vi "select gating.vi"() -> ()   [LabVIEW 2016]
doc: "Takes the pixie 4 values and creates a 2d spectrum based on the gate ROI and the desired spectrum"
uses:
  pixie2d/controls/energy 2d selection.ctl
  pixie2d/sub vi/chopper.ctl
  <vilib>/Utility/miscctls.llb/LVPointDoubleTypeDef.ctl
  controls/read write shift control.ctl
  <vilib>/DAQmx/write.llb/DAQmx Write (Digital Wfm 1Chan NSamp).vi
  <vilib>/Waveform/DWDTOps.llb/DWDT Uncompress Digital.vi
  <vilib>/DAQmx/miscellaneous.llb/DAQmx Fill In Error Info.vi
  <vilib>/Waveform/DWDTOps.llb/DWDT Boolean Array to Digital.vi
  <vilib>/DAQmx/configure/timing.llb/DAQmx Timing (Burst Import Clock).vi
  <vilib>/Waveform/DWDTOps.llb/DWDT Append Digital Samples.vi
  <resource>/objmgr/daqmx.rc
  <vilib>/Analysis/NI_AALPro.lvlib
panel:
  out "Chopper gain error":errorcluster
  in  "Tab Control":T1(tab)
  in  "stop":bool
  in  "set gate":bool
  in  "reset spectrum":bool
  in  "which spectrum":string(combo)="full spectrum pulser"
  in  "gate change":bool
  out "2d display":u64[][](graph) caption="full spectrum"
  in  "save image":bool
  out "2d gate active?":bool
  out "X Peak":i32
  out "Y peak":i32
  in  "na/V":dbl=1000.0
  in  "Energy 2d gate":T2="1 vs 2"
  in  "channel":string(combo)="Channel 1"
  out "MCA Histograms":u32[][](graph)
  in  "gain":i32=10 min=1 max=100 step=1
  in  "beam chopper":T3
  out "data":string
  out "task done?":bool
  out "location":dbl
  out "peak":dbl
  out "fwhm":i32
  in  "Module number":u16
  in  "reset count rate (cps)":i32=500000
  out "Loop iterations":i32
  out "std percent":dbl format="%0.2f"
  in  "chopper gain":i32(slide)=50 scale=0.0..20.0
  out "digital data out 3":digitaldata
  out "digital data out 2":digitaldata
  out "output waveform 3":digitalwaveform(waveform)={"t0"=timestamp(0 s since 1904-01-01), "dt"=1.0, "Y"={"transitions"=[], "data"=[]}}
  out "output waveform 2":digitalwaveform(waveform)={"t0"=timestamp(0 s since 1904-01-01), "dt"=1.0, "Y"={"transitions"=[], "data"=[]}}
  out "20UA_Chop_Tune.hws":digitalwaveform(waveform)={"t0"=timestamp(0 s since 1904-01-01), "dt"=1e-06, "Y"={"transitions"=[], "data"=array100000x16[1600000 elements]}}
  out "MCA Histogram cursor error":errorcluster
  out "Chopper error":errorcluster
  out "Tune Stable to Detector Error":errorcluster
  out "Chopper Pulse Creation error":errorcluster
  out "Chopped Current SV error":errorcluster
  out "DAQmx task end error 2":errorcluster
  out "DAQmx task end error 1":errorcluster
  out "Stop/Chopper Variant conversion":errorcluster
  out "Tune Stable DAQmx write error":errorcluster
  in  "chopper factor":u32(knob)=5 scale=0.0..10.0
  # "Directions\n1) select which spectrum \n     and 2d gate you want\n     to  view\n\n2)  When the ROI is located\n      double click on\n      chart to start\n      drawing gate\n\n3)   When gate is drawn,\n      double click the mouse to \n      stop the gate from being\n      drawn.  press gate \n       change and set gate will\n      appear\n\n4)   press set gate, and\n      gate will be generated\n\n5)  Once the gate is drawn,\n      make sure it covers the \n      region that you want\n      defined\n\n6)  To view gate, right click\n      on graph and select view\n     gates."
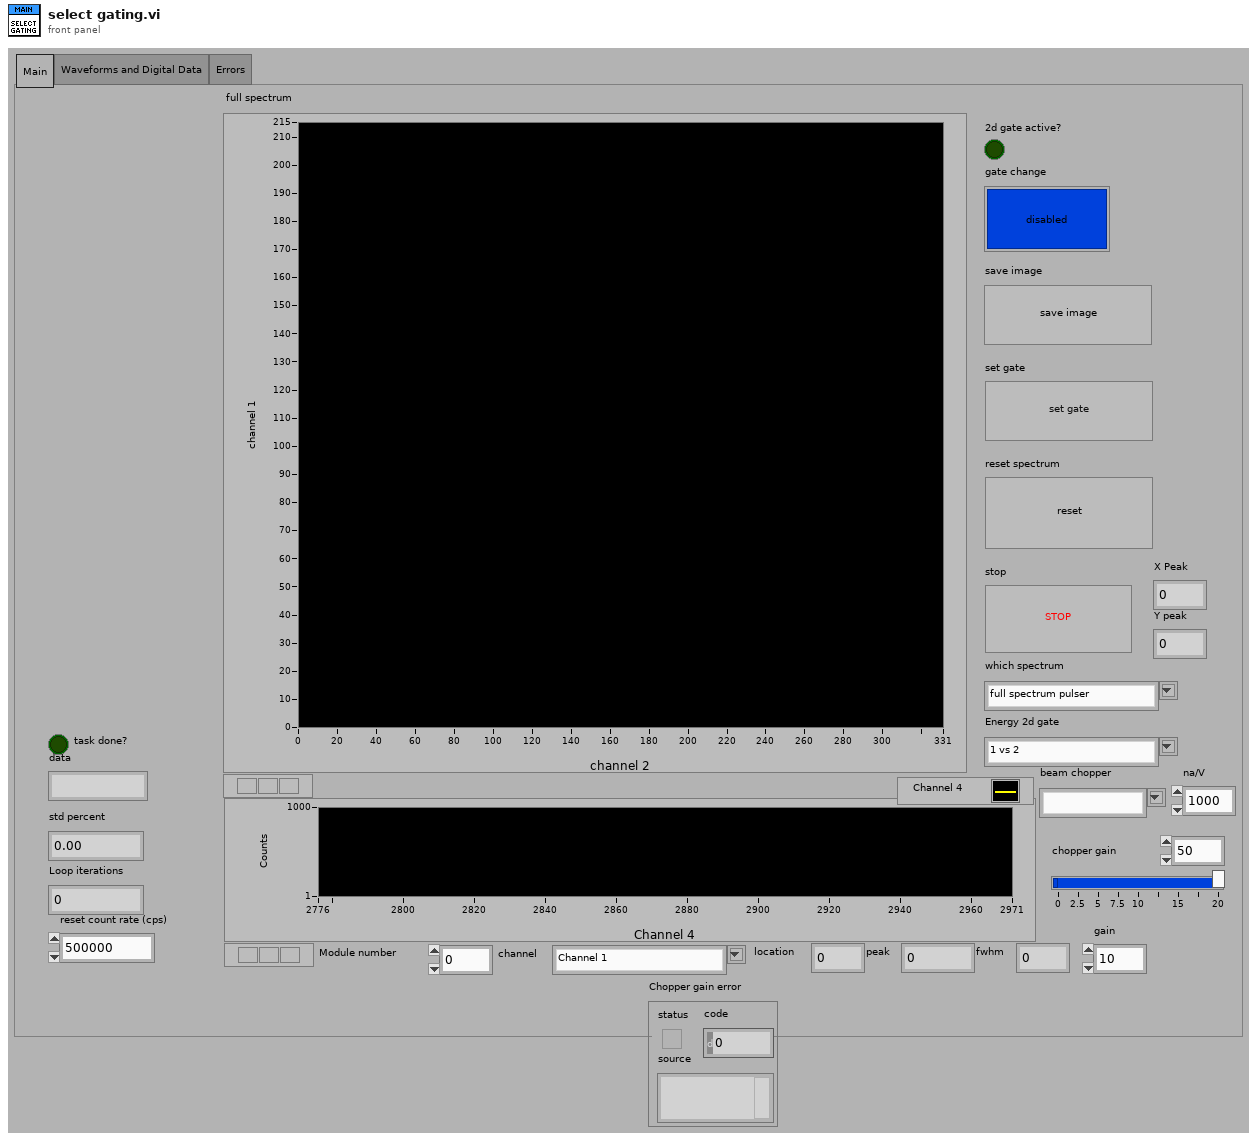
[diagram p1: front panel]
types:
  T1 = enum32{"Main", "Waveforms and Digital Data", "Errors"}
  T2 = typedef "energy 2d selection.ctl" = string
  T3 = typedef "chopper.ctl" = string
  T4 = typedef "LVPointDoubleTypeDef.ctl" = cluster{"X":dbl, "Y":dbl}
  T5 = typedef "read write shift control.ctl" = string
  T6 = typedef "LVPoint32TypeDef.ctl" = cluster{"Horizontal":i32, "Vertical":i32}
  T7 = typedef "imagedata.ctl" = cluster{"image type":i32, "image depth":i32, "image":u8[], "mask":u8[], "colors":u32[], "Rectangle":cluster{"left":i16, "top":i16, "right":i16, "bottom":i16}}
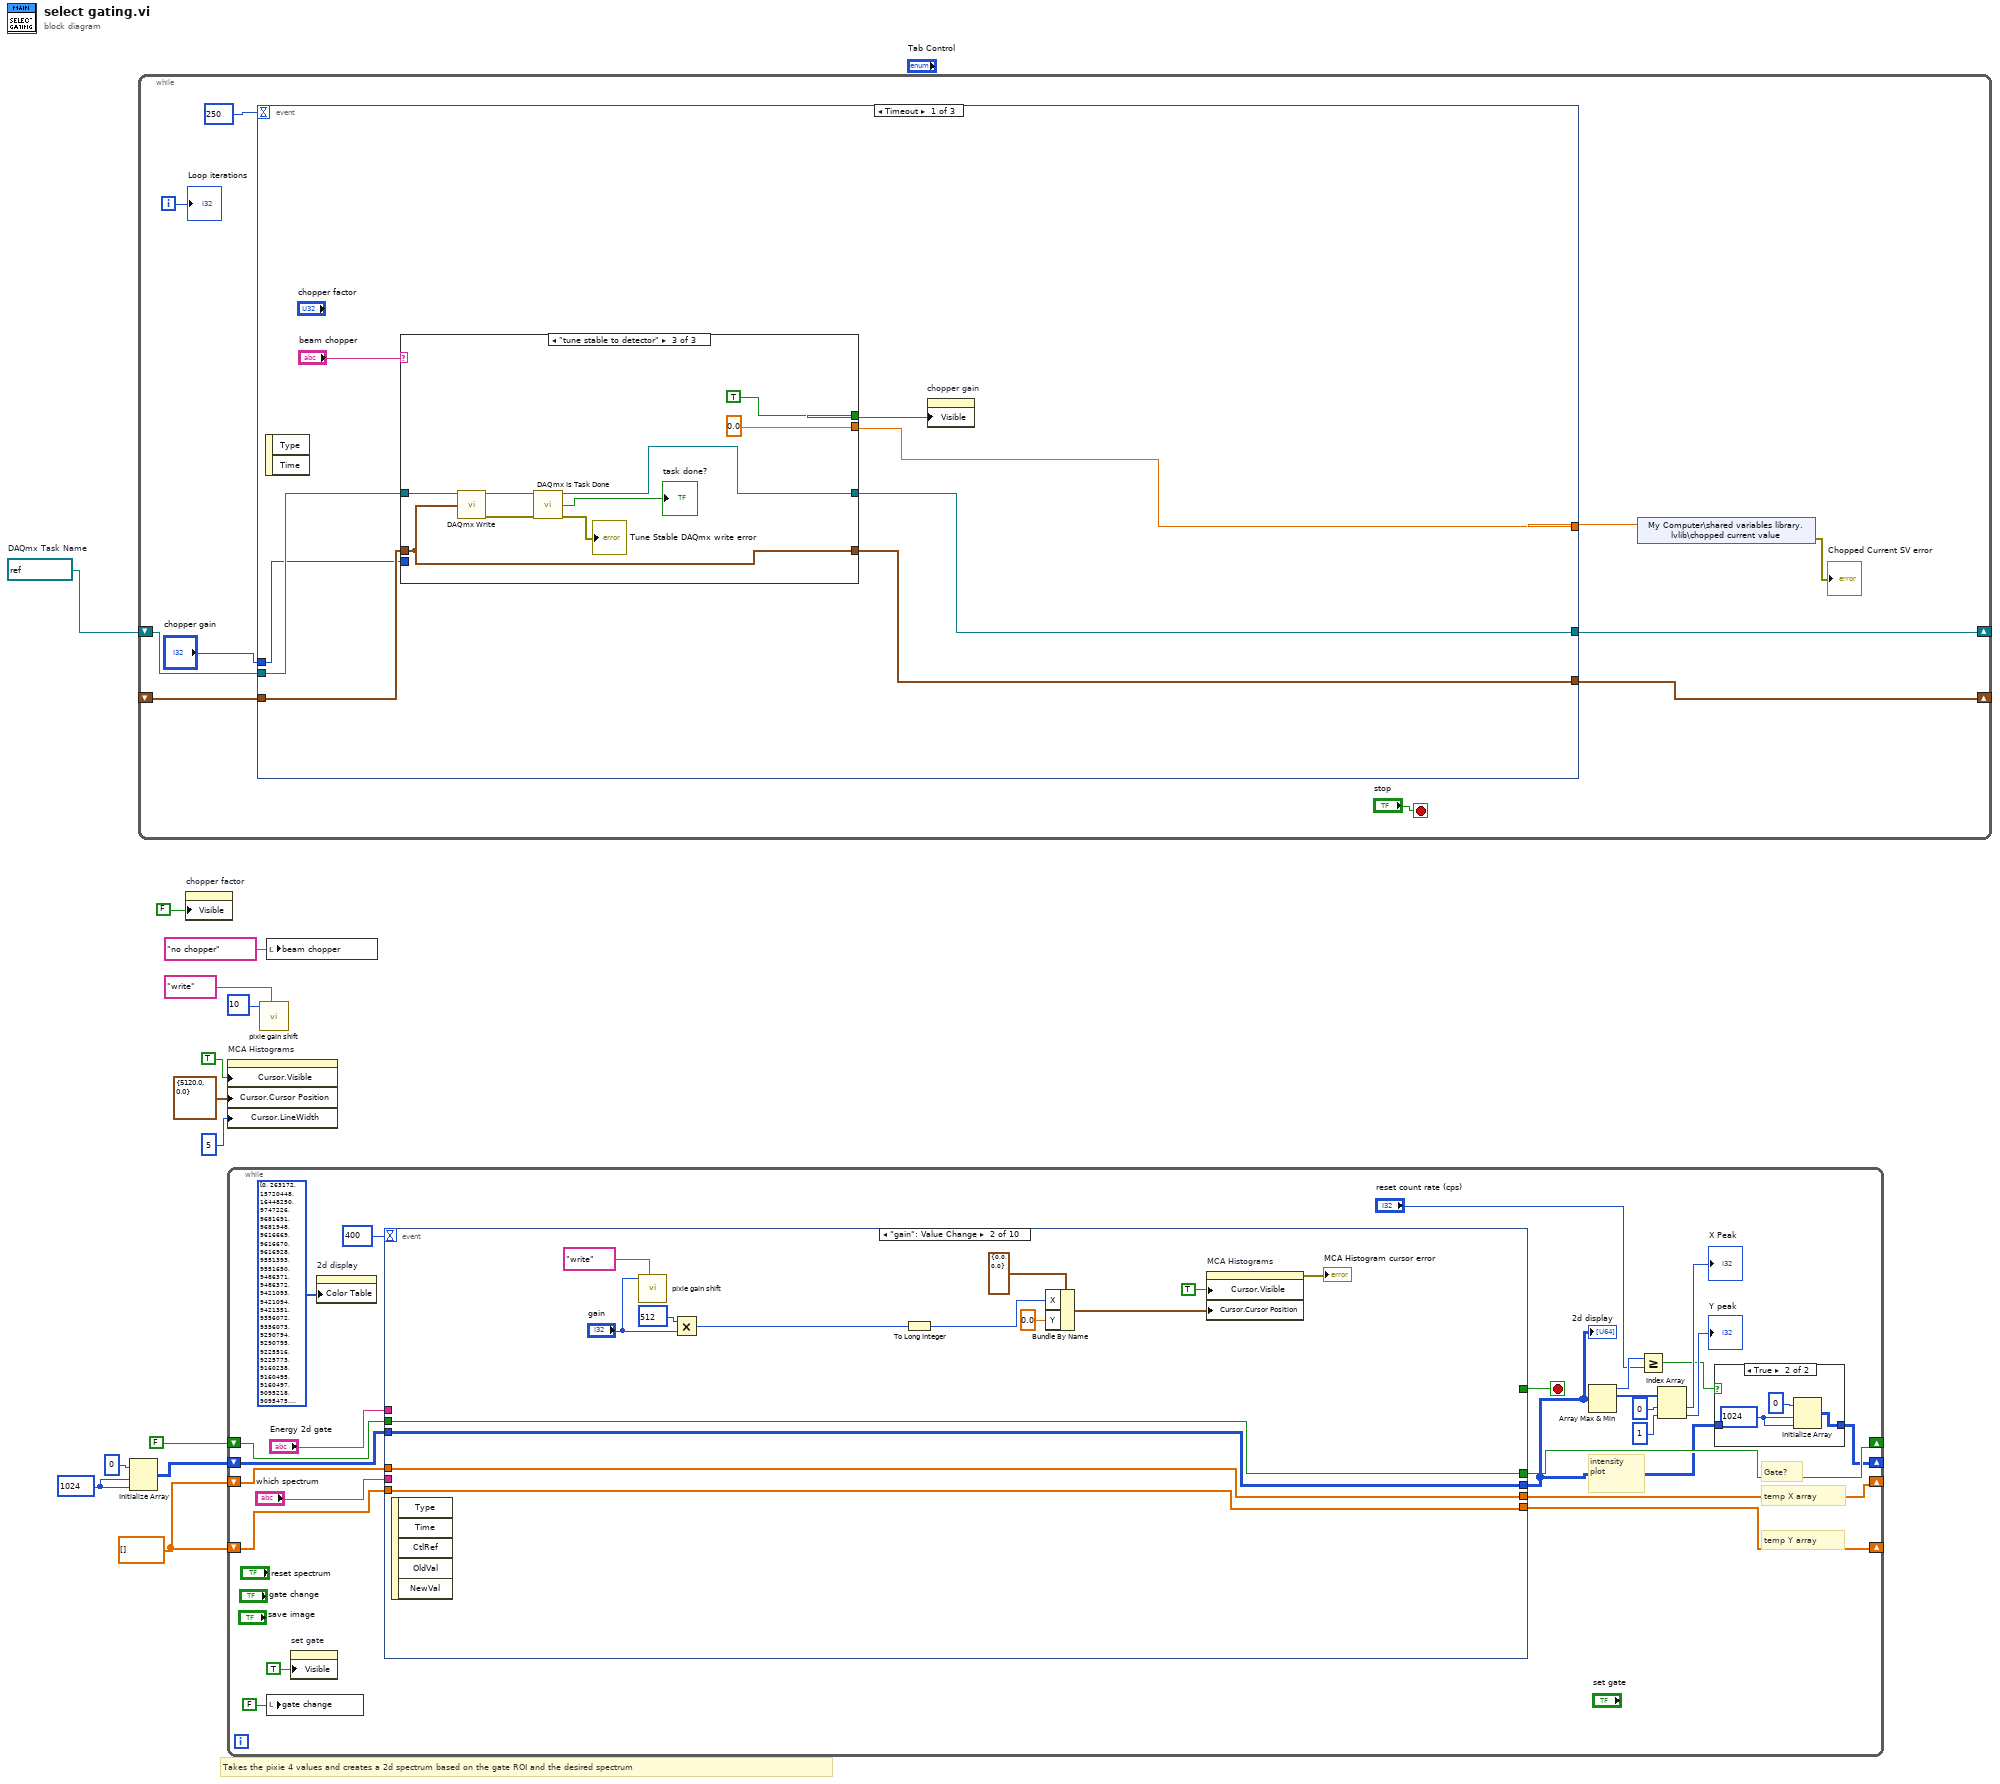
[diagram p0: block diagram]
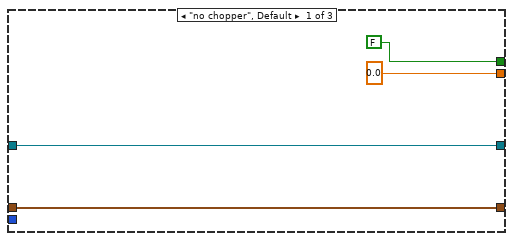
[diagram p2: hidden frame]
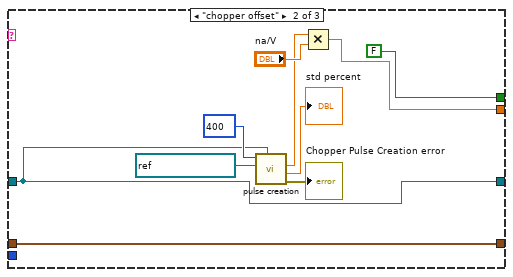
[diagram p3: hidden frame]
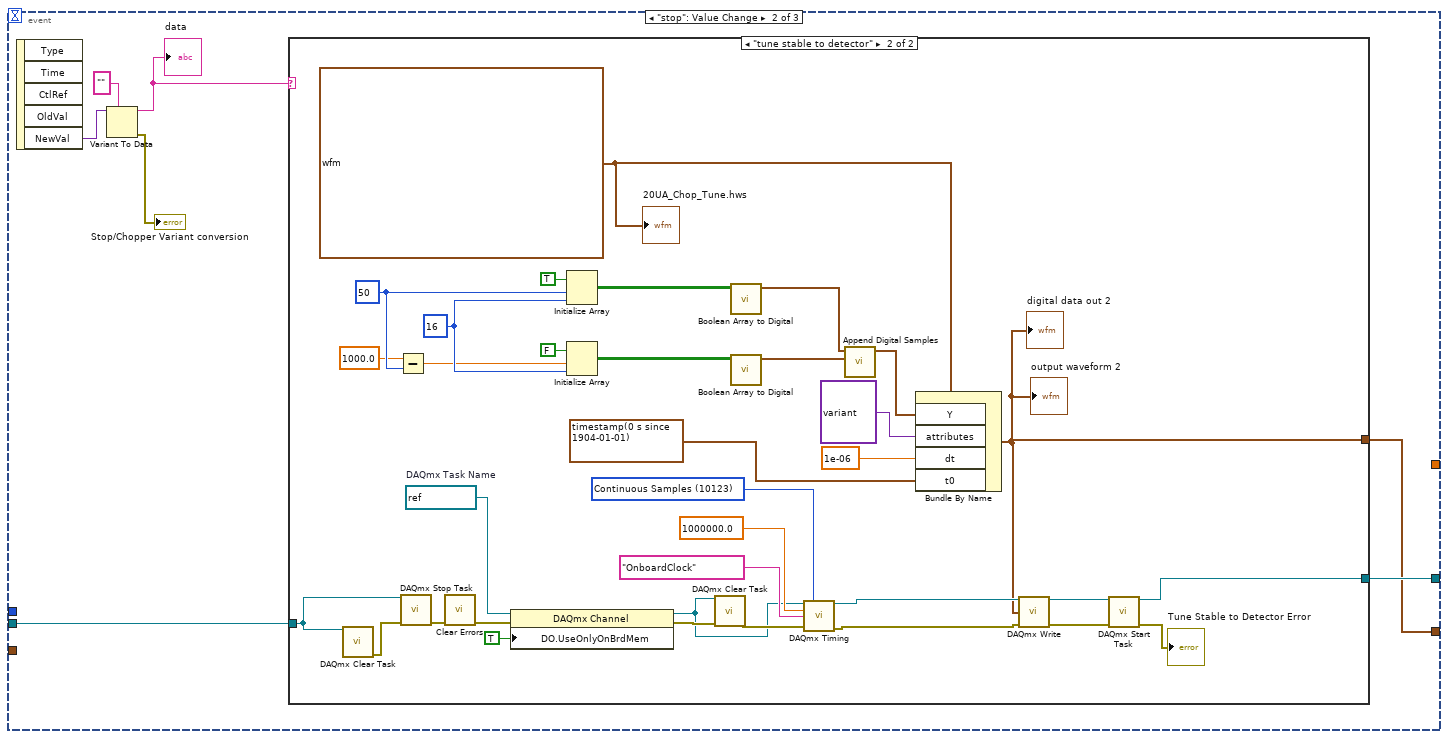
[diagram p4: hidden frame]
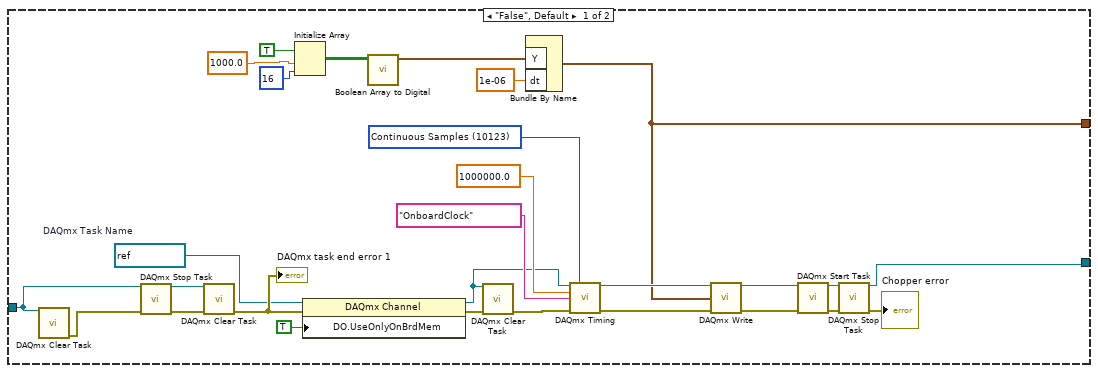
[diagram p5: hidden frame]
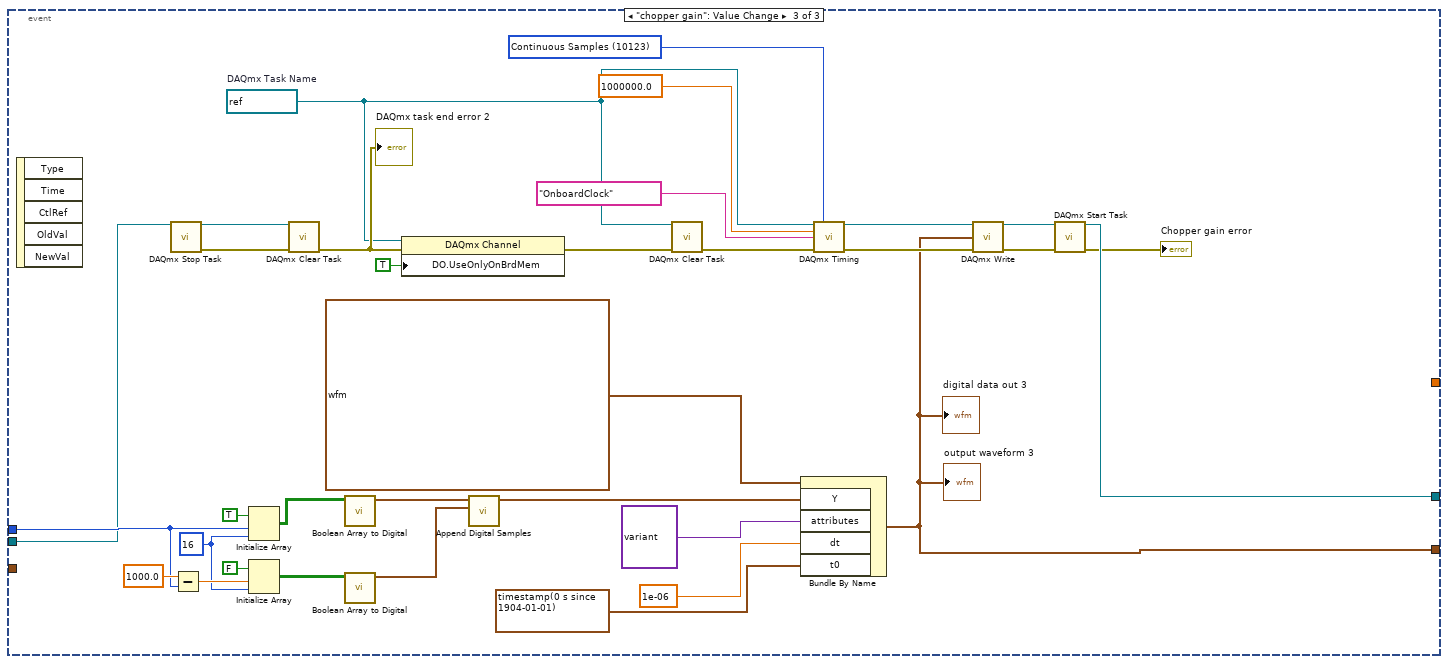
[diagram p6: hidden frame]
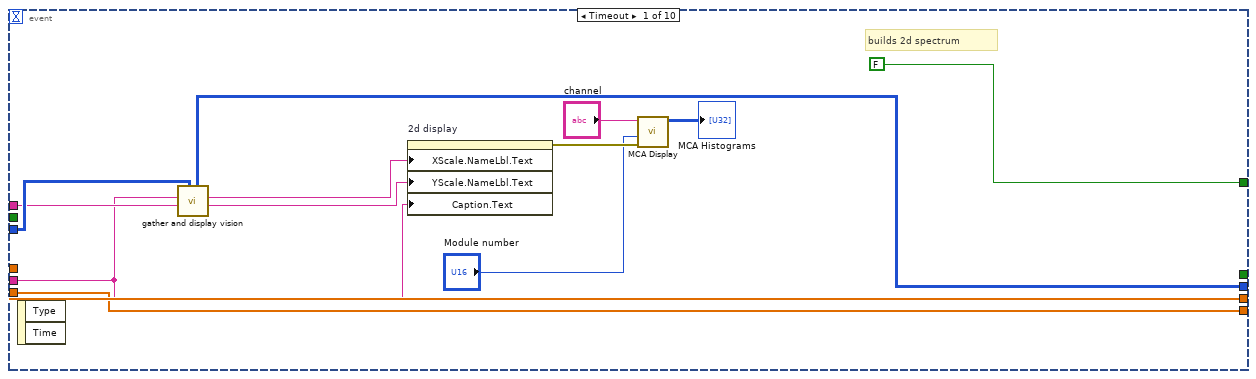
[diagram p8: hidden frame]
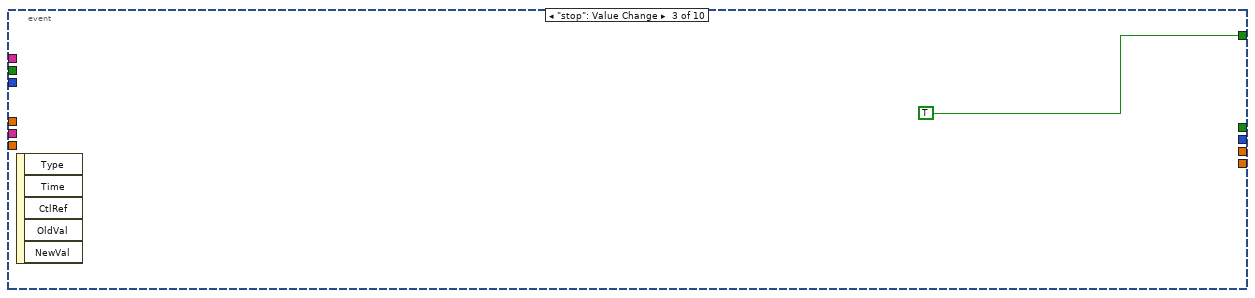
[diagram p9: hidden frame]
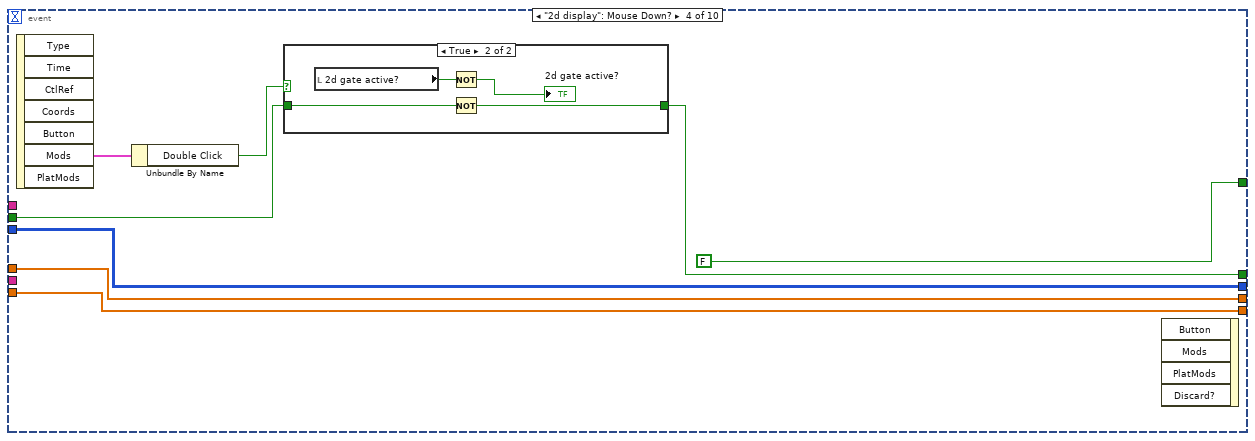
[diagram p10: hidden frame]
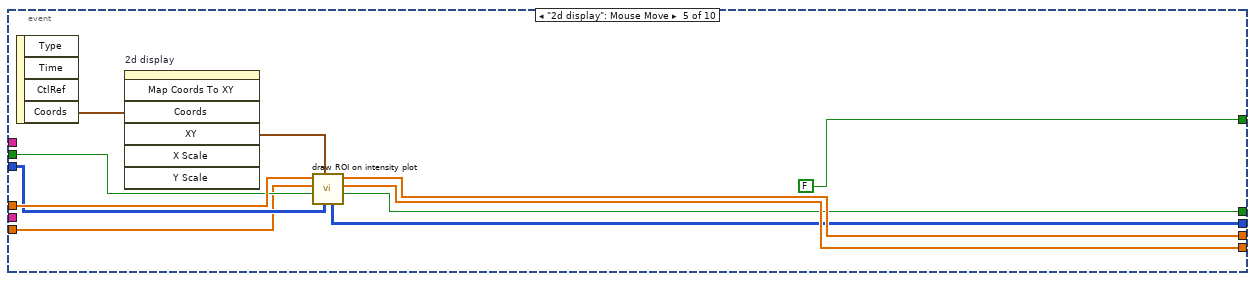
[diagram p12: hidden frame]
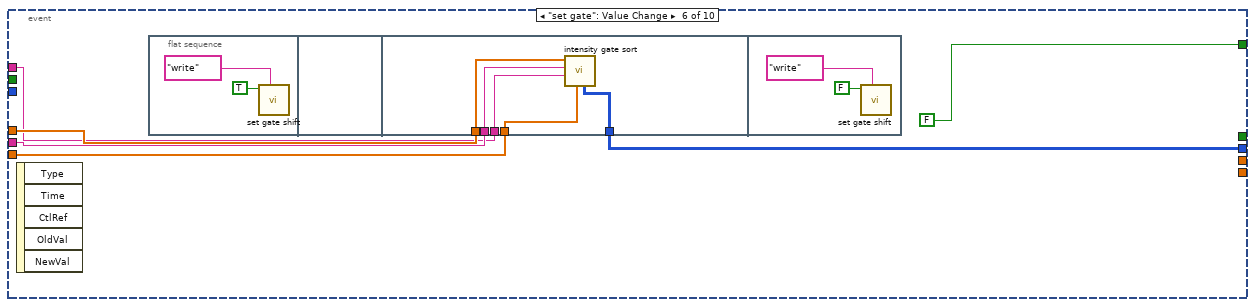
[diagram p13: hidden frame]
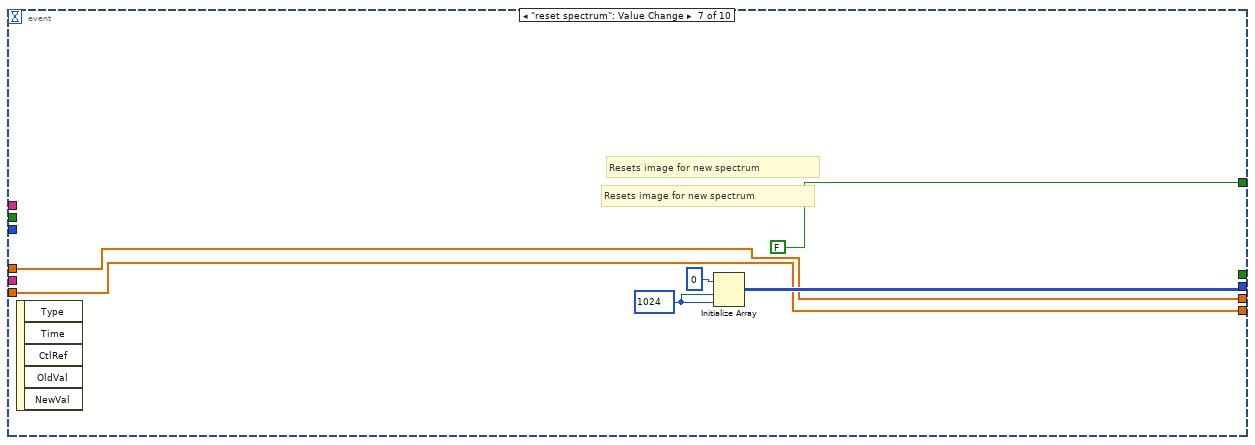
[diagram p14: hidden frame]
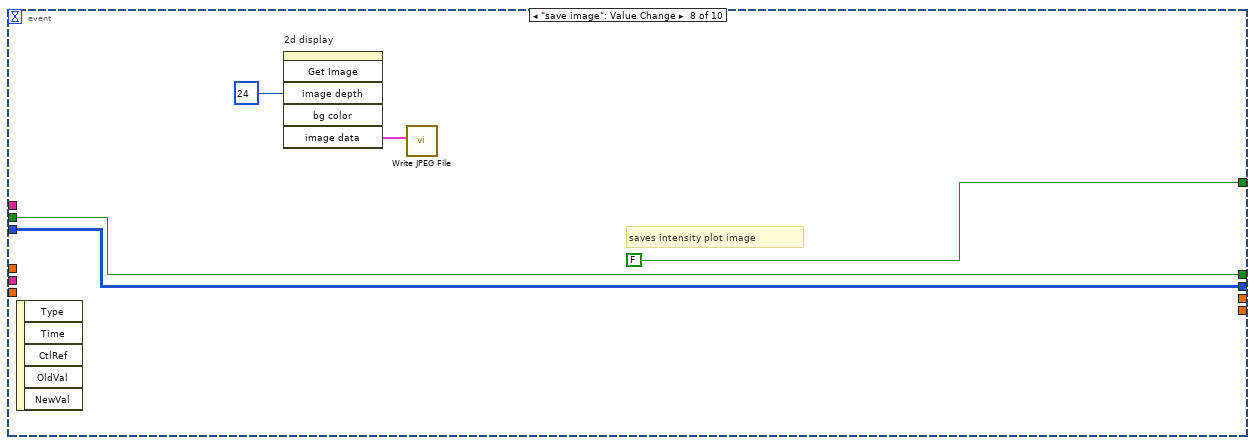
[diagram p15: hidden frame]
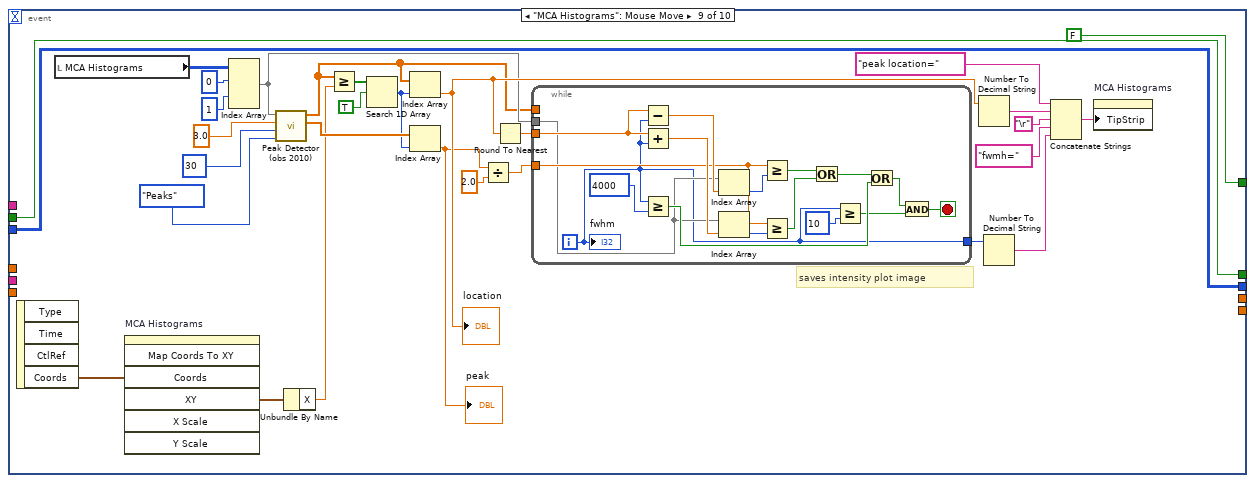
[diagram p16: hidden frame]
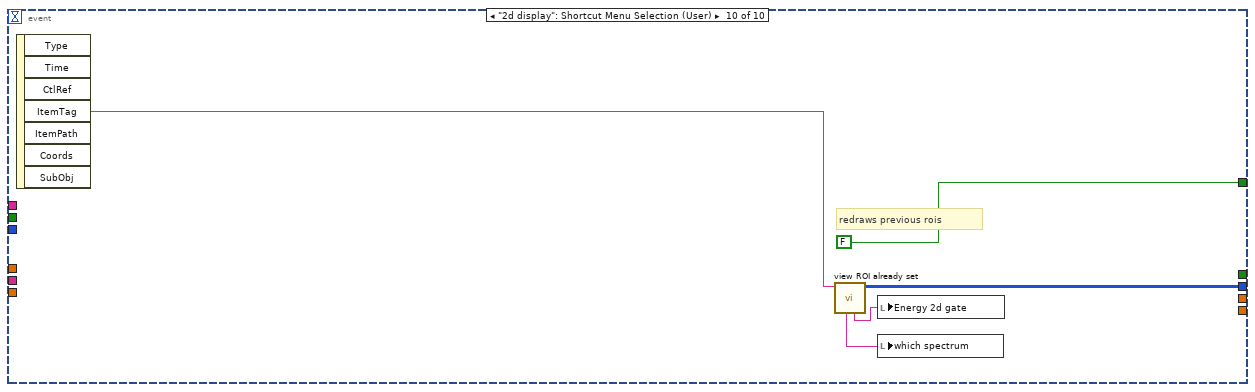
[diagram p17: hidden frame]
diagram:
  w1 = refnum<k21> "chop2"  # DAQmx Task Name
  w9 = dbl[] []
  w13 = u64 1024
  # "Takes the pixie 4 values and creates a 2d spectrum based on the gate ROI and the desired spectrum"
  n1 = Initialize Array(u64 0 ("X Resolution"), w13, w13) -> (w11:u64[][])
  n2 = while {
    shift-right: [w19] -> _
    shift-left: _ -> [w18]
    shift-right: [w16] -> _
    shift-left: w1 -> [w22]
    i -> [w15]
    stop <- "stop" stop-if-true
    n3 = event shown="[0] Timeout" {
      selector: _ -> [_ _ _]
      dyn-events: _ -> [_ _ _]
      timeout: 250 -> [_ _ _]
      tunnel: [w24 _ _] -> w23
      tunnel: w22 -> [w31 w58 w125]
      tunnel: [w29 w55 w128] -> w19
      tunnel: w18 -> [w30 _ _]
      tunnel: "chopper gain" -> [w25 _ w129]
      tunnel: [w28 w56 w126] -> w16
      event Timeout {
        n4 = event-data() -> ()  [unwired: 1 in, 2 out]
        n5 = case shown="\"tune stable to detector\"" "beam chopper" {
          tunnel: [0.0 w43 0.0] -> w24
          tunnel: w31 -> [w32 w37 w50]
          tunnel: [FALSE ("Visible") FALSE ("Visible") TRUE ("Visible")] -> w27
          tunnel: w30 -> [w33 w42 w49]
          tunnel: [w33 w42 w49] -> w29
          tunnel: [w32 w37 w46] -> w28
          tunnel: w25 -> [_ _ _]
          frame "no chopper", Default {
          }
          frame "chopper offset" {
            n6 = call "pulse creation.vi"("DAQmx Task Name"=w37, "task/channels in"=refnum<k21> "testcurrent", "chopper width(usec)"=u32 400) -> ("error out"=→"Chopper Pulse Creation error":errorcluster, "std percent"=→"std percent":dbl, "mean"=w41:dbl)  [unwired: 4 in, 2 out]
            n7 = Multiply(x=w41, y="na/V") -> (x*y=w43:dbl)
          }
          frame "tune stable to detector" {
            n8 = call-poly <vilib>:"DAQmx Write.vi"("task/channels in"=w50, "data"=w49) -> ("task out"=w48:refnum<k21>, "error out"=w47:errorcluster)  [unwired: 11 in, 1 out]
            n9 = call <vilib>:"DAQmx Is Task Done.vi"("task/channels in"=w48, "error in"=w47) -> ("task out"=w46:refnum<k21>, "task done?"=→"task done?":bool, "error out"=→"Tune Stable DAQmx write error":errorcluster)  [unwired: 11 in]
          }
        }
        n10 = property on="chopper gain" class="Slide (strict)"("Visible"=w27) -> ()  [unwired: 2 in, 2 out]
      }
      event "stop": Value Change {
        n11 = event-data() -> ("NewVal"=w61:variant)  [unwired: 1 in, 4 out]
        n12 = Variant To Data(type="", Variant=w61) -> (data=w57:string, error out=→"Stop/Chopper Variant conversion":errorcluster)  [unwired: 1 in]
        "data" <- w57
        n13 = case shown="\"tune stable to detector\"" w57 {
          tunnel: w58 -> [w67 w92]
          tunnel: [w68 w99] -> w55
          tunnel: [w63 w96] -> w56
          frame "False", Default {
            w74 = refnum<k21> "chop2"  # DAQmx Task Name
            w83 = 10123 items=["Finite Samples"=10178, "Continuous Samples"=10123, "Hardware Timed Single Point"=12522] ("sample mode")
            n14 = call <vilib>:"DAQmx Clear Task.vi"("task in"=w67) -> ("error out"=w66:errorcluster)  [unwired: 14 in]
            n15 = call <vilib>:"DAQmx Stop Task.vi"("task/channels in"=w67, "error in"=w66) -> ("task out"=w77:refnum<k21>, "error out"=w79:errorcluster)  [unwired: 12 in]
            n16 = call <vilib>:"DAQmx Clear Task.vi"("task in"=w77, "error in"=w79) -> ("error out"=w80:errorcluster)  [unwired: 13 in]
            "DAQmx task end error 1" <- w80
            n17 = Initialize Array(TRUE, 1000.0 ("x"), 16 ("dimension size")) -> (w86:bool[][])
            n18 = property class="DAQmx Channel"(reference=w74, error in=w80, "DO.UseOnlyOnBrdMem"=TRUE) -> (reference out=w69:refnum<k21>, error out=w73:errorcluster)
            n19 = call-poly <vilib>:"Boolean Array to Digital.vi"("boolean array"=w86) -> ("digital waveform"=w85:digitalwaveform)  [unwired: 9 in, 1 out]
            n20 = call <vilib>:"DAQmx Clear Task.vi"("task in"=w69, "error in"=w73) -> ("error out"=w72:errorcluster)  [unwired: 13 in]
            n21 = Bundle By Name("Y"=w85, "dt"=1e-06) -> (w68:digitalwaveform)  [unwired: 1 in]
            n22 = call-poly <vilib>:"DAQmx Timing.vi"("task/channels in"=w69, "sample mode"=w83, "sample clock rate"=1000000.0 ("rate"), "sample clock source"=tag "OnboardClock", "error in"=w72) -> ("task out"=w75:refnum<k21>, "error out"=w76:errorcluster)  [unwired: 9 in]
            n23 = call-poly <vilib>:"DAQmx Write.vi"("task/channels in"=w75, "data"=w68, "error in"=w76) -> ("task out"=w82:refnum<k21>, "error out"=w81:errorcluster)  [unwired: 10 in, 1 out]
            n24 = call <vilib>:"DAQmx Start Task.vi"("task/channels in"=w82, "error in"=w81) -> ("task out"=w65:refnum<k21>, "error out"=w64:errorcluster)  [unwired: 12 in]
            n25 = call <vilib>:"DAQmx Stop Task.vi"("task/channels in"=w65, "error in"=w64) -> ("task out"=w63:refnum<k21>, "error out"=→"Chopper error":errorcluster)  [unwired: 12 in]
          }
          frame "tune stable to detector" {
            w110 = 50 ("dimension size 2")
            w119 = 16 ("dimension size")
            w101 = digitalwaveform {"t0"=timestamp(0 s since 1904-01-01), "dt"=1e-06, "Y"={"transitions"=[], "data"=array100000x16[1600000 elements]}} ("20UA_Chop_Tune.hws")
            w105 = 10123 items=["Finite Samples"=10178, "Continuous Samples"=10123, "Hardware Timed Single Point"=12522] ("sample mode")
            w103 = refnum<k21> "chop2"  # DAQmx Task Name
            n26 = call <vilib>:"DAQmx Clear Task.vi"("task in"=w92) -> ("error out"=w91:errorcluster)  [unwired: 14 in]
            n27 = Subtract(x=1000.0, y=w110) -> (x-y=w111:dbl)
            n28 = call <vilib>:"DAQmx Stop Task.vi"("task/channels in"=w92, "error in"=w91) -> ("error out"=w90:errorcluster)  [unwired: 12 in, 1 out]
            n29 = call <vilib>:"Clear Errors.vi"("error in (no error)"=w90) -> ("error out"=w93:errorcluster)  [unwired: 5 in, 1 out]
            n30 = property class="DAQmx Channel"(reference=w103, error in=w93, "DO.UseOnlyOnBrdMem"=TRUE) -> (reference out=w95:refnum<k21>, error out=w98:errorcluster)
            n31 = Initialize Array(TRUE, w110, w119) -> (w120:bool[][])
            n32 = Initialize Array(FALSE, w111, w119) -> (w121:bool[][])
            n33 = call <vilib>:"DAQmx Clear Task.vi"("task in"=w95, "error in"=w98) -> ("error out"=w97:errorcluster)  [unwired: 13 in]
            n34 = call-poly <vilib>:"Boolean Array to Digital.vi"("boolean array"=w120) -> ("digital waveform"=w118:digitalwaveform)  [unwired: 9 in, 1 out]
            n35 = call-poly <vilib>:"Boolean Array to Digital.vi"("boolean array"=w121) -> ("digital waveform"=w113:digitalwaveform)  [unwired: 9 in, 1 out]
            n36 = call-poly <vilib>:"DAQmx Timing.vi"("task/channels in"=w95, "sample mode"=w105, "sample clock rate"=1000000.0 ("rate"), "sample clock source"=tag "OnboardClock", "error in"=w97) -> ("task out"=w106:refnum<k21>, "error out"=w107:errorcluster)  [unwired: 9 in]
            n37 = call-poly <vilib>:"Append Digital Samples.vi"("digital waveform B"=w113, "digital waveform A"=w118) -> ("digital waveform out"=w122:digitalwaveform)  [unwired: 8 in, 1 out]
            n38 = Bundle By Name(cluster=w101, "Y"=w122, "attributes"=variant, "dt"=1e-06, "t0"=timestamp(0 s since 1904-01-01)) -> (w99:digitalwaveform)
            "digital data out 2" <- w99
            "output waveform 2" <- w99
            n39 = call-poly <vilib>:"DAQmx Write.vi"("task/channels in"=w106, "data"=w99, "error in"=w107) -> ("task out"=w109:refnum<k21>, "error out"=w108:errorcluster)  [unwired: 10 in, 1 out]
            n40 = call <vilib>:"DAQmx Start Task.vi"("task/channels in"=w109, "error in"=w108) -> ("task out"=w96:refnum<k21>, "error out"=→"Tune Stable to Detector Error":errorcluster)  [unwired: 12 in]
            "20UA_Chop_Tune.hws" <- w101
          }
        }
      }
      event "chopper gain": Value Change {
        w134 = 16 ("dimension size")
        w148 = 10123 items=["Finite Samples"=10178, "Continuous Samples"=10123, "Hardware Timed Single Point"=12522] ("sample mode")
        w151 = refnum<k21> "chop2"  # DAQmx Task Name
        n41 = event-data() -> ()  [unwired: 1 in, 5 out]
        n42 = call <vilib>:"DAQmx Stop Task.vi"("task/channels in"=w125) -> ("task out"=w155:refnum<k21>, "error out"=w154:errorcluster)  [unwired: 13 in]
        n43 = Subtract(x=1000.0, y=w129) -> (x-y=w142:dbl)
        n44 = Initialize Array(TRUE, w129, w134) -> (w133:bool[][])
        n45 = Initialize Array(FALSE, w142, w134) -> (w132:bool[][])
        n46 = call <vilib>:"DAQmx Clear Task.vi"("task in"=w155, "error in"=w154) -> ("error out"=w156:errorcluster)  [unwired: 13 in]
        "DAQmx task end error 2" <- w156
        n47 = call-poly <vilib>:"Boolean Array to Digital.vi"("boolean array"=w133) -> ("digital waveform"=w135:digitalwaveform)  [unwired: 9 in, 1 out]
        n48 = call-poly <vilib>:"Boolean Array to Digital.vi"("boolean array"=w132) -> ("digital waveform"=w140:digitalwaveform)  [unwired: 9 in, 1 out]
        n49 = property class="DAQmx Channel"(reference=w151, error in=w156, "DO.UseOnlyOnBrdMem"=TRUE) -> (error out=w150:errorcluster)  [unwired: 1 out]
        n50 = call-poly <vilib>:"Append Digital Samples.vi"("digital waveform B"=w140, "digital waveform A"=w135) -> ("digital waveform out"=w131:digitalwaveform)  [unwired: 8 in, 1 out]
        n51 = call <vilib>:"DAQmx Clear Task.vi"("task in"=w151, "error in"=w150) -> ("error out"=w153:errorcluster)  [unwired: 13 in]
        n52 = Bundle By Name(cluster=digitalwaveform {"t0"=timestamp(0 s since 1904-01-01), "dt"=1e-06, "Y"={"transitions"=[], "data"=array100000x16[1600000 elements]}} ("20UA_Chop_Tune.hws"), "Y"=w131, "attributes"=variant, "dt"=1e-06, "t0"=timestamp(0 s since 1904-01-01)) -> (w128:digitalwaveform)
        "digital data out 3" <- w128
        "output waveform 3" <- w128
        n53 = call-poly <vilib>:"DAQmx Timing.vi"("task/channels in"=w151, "sample mode"=w148, "sample clock rate"=1000000.0 ("rate"), "sample clock source"=tag "OnboardClock", "error in"=w153) -> ("task out"=w147:refnum<k21>, "error out"=w146:errorcluster)  [unwired: 9 in]
        n54 = call-poly <vilib>:"DAQmx Write.vi"("task/channels in"=w147, "data"=w128, "error in"=w146) -> ("task out"=w144:refnum<k21>, "error out"=w145:errorcluster)  [unwired: 10 in, 1 out]
        n55 = call <vilib>:"DAQmx Start Task.vi"("task/channels in"=w144, "error in"=w145) -> ("task out"=w126:refnum<k21>, "error out"=→"Chopper gain error":errorcluster)  [unwired: 12 in]
      }
    }
    n56 = shared-variable "My Computer\\shared variables library.lvlib\\chopped current value"(w23) -> (error out=→"Chopped Current SV error":errorcluster)  [unwired: 1 in]
    "Loop iterations" <- w15
  }
  n57 = property on="chopper factor" class="Knob (strict)"("Visible"=FALSE) -> ()  [unwired: 2 in, 2 out]
  n58 = property on="MCA Histograms" class="WFGraph (strict)"("Cursor.Visible"=TRUE, "Cursor.Cursor Position"=T4 {"X"=5120.0, "Y"=0.0}, "Cursor.LineWidth"=u8 5 ("Cursor.Line Width")) -> ()  [unwired: 2 in, 2 out]
  n59 = while {
    shift-right: [w157] -> _
    shift-left: w11 -> [w177]
    shift-right: [w175] -> _
    shift-left: FALSE -> [w174]
    shift-right: [w170] -> _
    shift-left: w9 -> [w172]
    shift-right: [w171] -> _
    shift-left: w9 -> [w173]
    stop <- w162 stop-if-true
    # "intensity\nplot"
    # "Gate?"
    # "temp Y array"
    # "temp X array"
    n60 = local write "gate change"(FALSE ("gate change")) -> ()
    n61 = property on="set gate" class="Bool"("Visible"=TRUE) -> ()  [unwired: 2 in, 2 out]
    n62 = property on="2d display" class="IntGraph (strict)"("Color Table"=u32[] [0, 263172, 15720448, 16448250, 9747226, 9681691, 9681948, 9616669, 9616670, 9616928, 9551393, 9551650, 9486371, 9486372, 9421093, 9421094, 9421351, 9356072, 9356073, 9290794, 9290795, 9225516, 9225773, 9160238, 9160495, 9160497, 9095218, 9095475, 9029940, 9030197, 8964918, 8964919, 8965176, 8899641, 8899898, 8834619, 8834620, 8769341, 8769342, 8769599, 8704321, 8704322, 8639043, 8639044, 8573765, 8574022, 8574023, 8508744, 8508745, 8443466, 8443723, 8378188, 8378445, 8312910, 8313167, 8312912, 8247122, 8246867, 8181076, 8181077, 8115286, 8115031, 8114776, 8048985, 8048730, 7982939, 7982684, 7916893, 7916894, 7916639, 7850848, 7850594, 7784803, 7784548, 7718757, 7718502, 7718503, 7652712, 7652457, 7586666, 7586411, 7520620, 7520365, 7454574, 7454319, 7454320, 7388529, 7388275, 7322484, 7322229, 7256438, 7256183, 7255928, 7190137, 7190138, 7124347, 7124092, 7058301, 7058046, 7057791, 6992000, 6991745, 6926211, 6925956, 6860165, 6859910, 6859655, 6793864, 6793609, 6727818, 6727563, 6662028, 6661773, 6595982, 6595727, 6595472, 6529681, 6529426, 6463636, 6463381, 6397846, 6397591, 6397336, 6331545, 6331290, 6265499, 6265243, 6199451, 6199451, 6199195, 6133403, 6133147, 6067355, 6067100, 6001308, 6001052, 6000796, 5935260, 5935004, 5869212, 5868956, 5803164, 5802908, 5737116, 5736860, 5736604, 5671068, 5670813, 5605021, 5604765, 5538973, 5538717, 5538461, 5472669, 5472413, 5406877, 5406621, 5340829, 5340573, 5340317, 5274525, 5274270, 5208478, 5208478, 5142686, 5142430, 5142174, 5076382, 5076126, 5010334, 5010078, 4944286, 4944286, 4878494, 4878238, 4877982, 4812191, 4811935, 4746143, 4745887, 4680095, 4680095, 4679839, 4614047, 4613791, 4547999, 4547743, 4481951, 4481695, 4678303, 4874656, 5005472, 5201824, 5398176, 5594528, 5790880, 5987232, 6183584, 6314656, 6511008, 6707360, 6903712, 7100064, 7230880, 7427233, 7623585, 7819937, 8016545, 8212897, 8409249, 8540065, 8736417, 8932769, 9129121, 9325473, 9456545, 9652897, 9849249, 10045601, 10241954, 10438306, 10634658, 10765474, 10961826, 11158434, 11354786, 11551138, 11681954, 11878306, 12074658, 12271010, 12467362, 12663714, 12860323, 12991139, 13187491, 13383843, 13580195, 13776547, 13907363, 14103715, 14300323, 14496675, 14693027, 14889379, 15085731, 15216547, 15412900, 15609252, 15805604, 16002212, 16133028, 16329380, 16525732, 16722084, 16711680, 16448250, 16448250, 16448250]) -> ()  [unwired: 2 in, 2 out]
    n63 = event shown="[1] \"gain\": Value Change" {
      selector: _ -> [_ _ _ _ _ _ _ _ _ _]
      dyn-events: _ -> [_ _ _ _ _ _ _ _ _ _]
      timeout: 400 -> [_ _ _ _ _ _ _ _ _ _]
      tunnel: "Energy 2d gate" -> [w192 _ _ _ _ w240 _ _ _ _]
      tunnel: "which spectrum" -> [w191 _ _ _ _ w241 _ _ _ _]
      tunnel: w177 -> [w197 w200 _ w218 w229 _ _ w260 w265 _]
      tunnel: [w186 w200 _ w218 w228 w238 w255 w260 w265 w313] -> w158
      tunnel: [_ w201 _ w220 w230 _ _ w259 w264 _] -> w175
      tunnel: w174 -> [_ w201 _ w219 w231 _ _ w259 w264 _]
      tunnel: [w196 w203 _ w216 w234 _ w254 _ _ _] -> w171
      tunnel: [w195 w202 _ w217 w233 _ w253 _ _ _] -> w170
      tunnel: w173 -> [w196 w203 _ w216 w232 w242 w254 _ _ _]
      tunnel: w172 -> [w195 w202 _ w217 w227 w239 w253 _ _ _]
      tunnel: [FALSE ("Visible") _ TRUE ("Visible") FALSE ("Visible") FALSE ("Visible") FALSE ("Visible") FALSE ("Visible") FALSE ("Visible") FALSE ("Visible") FALSE ("Visible")] -> w162
      event Timeout {
        # "builds 2d spectrum"
        n64 = event-data() -> ()  [unwired: 1 in, 2 out]
        n65 = call "gather and display vision.vi"("intensity plot in"=w197, "Energy 2d gate"=w192, "which spectrum"=w191) -> ("Y Axis"=w193:string, "X Axis"=w194:string, "intensity plot out"=w186:i32[][])  [unwired: 5 in, 1 out]
        n66 = property on="2d display" class="IntGraph (strict)"("XScale.NameLbl.Text"=w194, "YScale.NameLbl.Text"=w193, "Caption.Text"=w191) -> (error out=w189:errorcluster)  [unwired: 2 in, 1 out]
        n67 = call "MCA Display.vi"("error in (no error)"=w189, "Module number"="Module number", "channel"="channel") -> ("MCA Histograms"=→"MCA Histograms":u32[][])  [unwired: 5 in, 3 out]
      }
      event "gain": Value Change {
        n68 = event-data() -> ()  [unwired: 1 in, 5 out]
        n69 = call "pixie gain shift.vi"("shift control"="write", "gain"="gain") -> ()  [unwired: 9 in, 1 out]
        n70 = Multiply(x=512 ("y"), y="gain") -> (x*y=w206:i32)
        n71 = To Long Integer(number=w206) -> (32bit integer=w205:i32)
        n72 = Bundle By Name(cluster=T4 {"X"=0.0, "Y"=0.0} ("Cursor.Cursor Position"), "X"=w205, "Y"=0.0) -> (w204:T4)
        n73 = property on="MCA Histograms" class="WFGraph (strict)"("Cursor.Visible"=TRUE, "Cursor.Cursor Position"=w204) -> (error out=→"MCA Histogram cursor error":errorcluster)  [unwired: 2 in, 1 out]
      }
      event "stop": Value Change {
        n74 = event-data() -> ()  [unwired: 1 in, 5 out]
      }
      event "2d display": Mouse Down? {
        n75 = event-data() -> ("Mods"=w214:cluster{"Double Click":bool, "Menu Key":bool})  [unwired: 1 in, 6 out]
        n76 = Unbundle By Name(w214) -> ("Double Click"=w215:bool)
        n77 = case shown="True" w215 {
          tunnel: [w221 w225] -> w220
          tunnel: w219 -> [w221 w224]
          frame False {
          }
          frame True {
            n78 = local read "2d gate active?"() -> (w222:bool)
            n79 = Not(x=w222) -> (.not. x?=→"2d gate active?":bool)
            n80 = Not(x=w224) -> (.not. x?=w225:bool)
          }
        }
        n81 = event-data() -> ()  [unwired: 5 in, 1 out]
      }
      event "2d display": Mouse Move {
        n82 = event-data() -> ("Coords"=w235:T6)  [unwired: 1 in, 3 out]
        n83 = invoke on="2d display" class="IntGraph (strict)" method="Map Coords To XY"("Coords"=w235) -> ("XY"=w236:cluster{"X":dbl, "Y":dbl})  [unwired: 6 in, 6 out]
        n84 = call "draw ROI on intensity plot.vi"("Intensity array in"=w229, "mouse positon"=w236, "draw gate? in"=w231, "y array in"=w227, "x array in"=w232) -> ("draw gate out"=w230:bool, "y array out"=w233:dbl[], "x array out"=w234:dbl[], "intensity array out"=w228:u64[][])  [unwired: 2 in, 1 out]
      }
      event "set gate": Value Change {
        n85 = event-data() -> ()  [unwired: 1 in, 5 out]
        n86 = flat-sequence {
          tunnel: w242 -> [w249]
          tunnel: w241 -> [w248]
          tunnel: w240 -> [w247]
          tunnel: w239 -> [w246]
          tunnel: [w245] -> w238
          frame #0 {
            n87 = call "set gate shift.vi"("read write"=T5 "write", "set gate In"=TRUE) -> ()  [unwired: 9 in, 1 out]
          }
          frame #1 {
          }
          frame #2 {
            n88 = call "intensity gate sort.vi"("Y array in"=w246, "Energy 2d gate"=w247, "which spectrum"=w248, "X array in"=w249) -> ("Intensity plot"=w245:u64[][])  [unwired: 6 in, 1 out]
          }
          frame #3 {
            n89 = call "set gate shift.vi"("read write"=T5 "write", "set gate In"=FALSE) -> ()  [unwired: 9 in, 1 out]
          }
        }
      }
      event "reset spectrum": Value Change {
        w256 = u64 1024
        # "Resets image for new spectrum"
        # "Resets image for new spectrum"
        n90 = event-data() -> ()  [unwired: 1 in, 5 out]
        n91 = Initialize Array(u64 0 ("X Resolution"), w256, w256) -> (w255:u64[][])
      }
      event "save image": Value Change {
        # "saves intensity plot image"
        n92 = event-data() -> ()  [unwired: 1 in, 5 out]
        n93 = invoke on="2d display" class="IntGraph (strict)" method="Get Image"("image depth"=24 ("Image Depth")) -> ("image data"=w261:T7)  [unwired: 5 in, 5 out]
        n94 = call <vilib>:"Write JPEG File.vi"("image data"=w261) -> ()  [unwired: 9 in, 2 out]
      }
      event "MCA Histograms": Mouse Move {
        # "saves intensity plot image"
        n95 = event-data() -> ("Coords"=w292:T6)  [unwired: 1 in, 3 out]
        n96 = local read "MCA Histograms"() -> (w267:u32[][])
        n97 = invoke on="MCA Histograms" class="WFGraph (strict)" method="Map Coords To XY"("Coords"=w292) -> ("XY"=w266:cluster{"X":dbl, "Y":dbl})  [unwired: 6 in, 6 out]
        n98 = Index Array(array=w267, index (row) #1=0 ("index (row)"), index (row) #2=1 ("disabled index (col)")) -> (element #1=w283:u32[])  [unwired: 2 in, 1 out]
        n99 = call <vilib>:"Peak Detector (obs 2010).vi"("peaks/valleys"=enum32{"Peaks", "Valleys"}."Peaks", "width"=30, "threshold"=3.0, "X"=w283) -> ("Amplitudes"=w278:dbl[], "Locations"=w277:dbl[])  [unwired: 3 in, 3 out]
        n100 = Unbundle By Name(w266) -> ("X"=w271:dbl)
        n101 = Greater Or Equal?(x=w277, y=w271) -> (x >= y?=w272:bool[])
        n102 = Search 1D Array(1D array=w272, element=TRUE) -> (index of element=w274:i32)  [unwired: 1 in]
        n103 = Index Array(array=w277, index=w274) -> (element=w285:dbl)
        "location" <- w285
        n104 = Index Array(array=w278, index=w274) -> (element=w281:dbl)
        "peak" <- w281
        n105 = Divide(x=w281, y=2.0) -> (x/y=w276:dbl)
        n106 = Round To Nearest(number=w285) -> (nearest integer value=w280:dbl)
        n107 = while {
          tunnel: w280 -> [w309]
          tunnel: w276 -> [w299]
          tunnel: w277 -> [_]
          tunnel: w283 -> [w294]
          tunnel: [w293] -> w290
          i -> [w293]
          stop <- w295 stop-if-true
          n108 = Subtract(x=w309, y=w293) -> (x-y=w307:dbl)
          n109 = Add(x=w309, y=w293) -> (x+y=w308:dbl)
          n110 = Greater Or Equal?(x=w293, y=4000) -> (x >= y?=w303:bool)
          n111 = Index Array(array=w294, index=w307) -> (element=w301:u32)
          n112 = Index Array(array=w294, index=w308) -> (element=w300:u32)
          n113 = Greater Or Equal?(x=w299, y=w301) -> (x >= y?=w306:bool)
          n114 = Greater Or Equal?(x=w299, y=w300) -> (x >= y?=w302:bool)
          n115 = Or(x=w306, y=w302) -> (x .or. y?=w304:bool)
          n116 = Greater Or Equal?(x=w293, y=10) -> (x >= y?=w296:bool)
          n117 = Or(x=w304, y=w303) -> (x .or. y?=w298:bool)
          n118 = And(x=w298, y=w296) -> (x .and. y?=w295:bool)
          "fwhm" <- w293
        }
        n119 = Number To Decimal String(number=w285) -> (decimal integer string=w286:string)  [unwired: 1 in]
        n120 = Number To Decimal String(number=w290) -> (decimal integer string=w289:string)  [unwired: 1 in]
        n121 = Concatenate Strings("peak location=" ("Tip Strip"), w286, "\r", "fwmh=" ("Tip Strip"), w289) -> (w291:string)
        n122 = property on="MCA Histograms" class="WFGraph (strict)"("TipStrip"=w291) -> ()  [unwired: 2 in, 2 out]
      }
      event "2d display": Shortcut Menu Selection (User) {
        # "redraws previous rois"
        n123 = event-data() -> ("ItemTag"=w314:string)  [unwired: 1 in, 6 out]
        n124 = call "view ROI already set.vi"("ItemTag"=w314) -> ("intensity plot"=w313:u64[][], "Energy 2d gate out"=w312:T2, "which spectrum"=w311:string)  [unwired: 7 in, 1 out]
        n125 = local write "Energy 2d gate"(w312) -> ()
        n126 = local write "which spectrum"(w311) -> ()
      }
    }
    "2d display" <- w158
    n127 = Array Max & Min(array=w158) -> (max value=w161:u64, max index (indices)=w168:i32[])  [unwired: 2 out]
    n128 = Greater Or Equal?(x=w161, y="reset count rate (cps)") -> (x >= y?=w159:bool)
    n129 = Index Array(array=w168, index #1=0 ("index"), index #2=1 ("index")) -> (element #1=→"X Peak":i32, element #2=→"Y peak":i32)
    n130 = case shown="True" w159 {
      tunnel: w158 -> [w181 _]
      tunnel: [w181 w182] -> w157
      frame False {
      }
      frame True {
        w184 = u64 1024
        n131 = Initialize Array(u64 0 ("X Resolution"), w184, w184) -> (w182:u64[][])
      }
    }
  }
  n132 = call "pixie gain shift.vi"("shift control"="write", "gain"=10) -> ()  [unwired: 9 in, 1 out]
  n133 = local write "beam chopper"(T3 "no chopper" ("beam chopper")) -> ()
